vi "Build Interrupt Status Message.vi"(5 "State With Arguments":string, 7 "Arguments (\"\")":string) -> (6 "CSM Message String":string)   [LabVIEW 2017, in "Communicable State Machine.lvlib"]
doc: "#### Build Interrupt Status Message.vi\n\nConcatenates an interrupt status message. The format is as follows:\n\n Status >> Arguments -><interrupt>\n\n> [!NOTE] Message Concatenation API\n> This type of API does not directly send messages, it only concatenates message strings. The strings need to be incorporated into the CSM's state queue and then sent and executed in Parse State Queue++.vi.\n> If you are familiar with CSM rules, you can skip using this type of API and directly type the corresponding message strings and operation strings in the text.\n\n\n<b>Controls</b>\n- <b>State with Arguments</b>: CSM interrupt status message string.\n- <b>Arguments (\"\")</b>: Argument information. Arguments included in <b>State with Arguments</b> will be replaced.\n\n<b>Indicators</b>\n- <b>CSM Message String</b>: The concatenated CSM message string."
uses:
  Communicable State Machine.lvlib
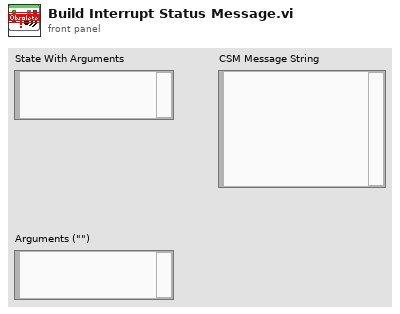
[diagram p1: front panel]
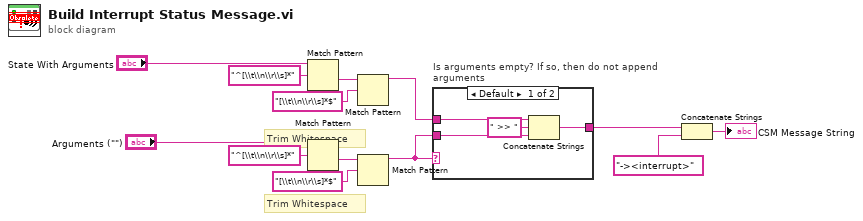
[diagram p0: block diagram]
diagram:
  # "Trim Whitespace"
  # "Trim Whitespace"
  n1 = Match Pattern(string="State With Arguments", regular expression="^[\\t\\n\\r\\s]*") -> (after substring=w6:string)  [unwired: 1 in, 3 out]
  n2 = Match Pattern(string="Arguments (\"\")", regular expression="^[\\t\\n\\r\\s]*") -> (after substring=w12:string)  [unwired: 1 in, 3 out]
  n3 = Match Pattern(string=w6, regular expression="[\\t\\n\\r\\s]*$") -> (before substring=w4:string)  [unwired: 1 in, 3 out]
  n4 = Match Pattern(string=w12, regular expression="[\\t\\n\\r\\s]*$") -> (before substring=w9:string)  [unwired: 1 in, 3 out]
  n5 = case "Is arguments empty? If so, then do not append arguments" shown="Default" w9 {
    tunnel: [w14 w18] -> w10
    tunnel: w4 -> [w17 w18]
    tunnel: w9 -> [w15 _]
    frame Default {
      n6 = Concatenate Strings(w17, " >> " ("string"), w15) -> (w14:string)
    }
    frame "" {
    }
  }
  n7 = Concatenate Strings(w10, "-><interrupt>" ("string")) -> (→"CSM Message String":string)
